vi "AOVoltageDAQmxGenWaveformBufferGeneration.vi"(0 "task/channels in":refnum<k21>, 1 "Samples per Buffer":dbl=1000.0, 3 "Amplitude":dbl=2.0 format="%0.2p", 5 "Desired Frequency":dbl=1000.0 format="%.2f", 7 "Waveform Type":T1(ring), 11 "error in (no error)":errorcluster, 12 "Cycles per Buffer":dbl=1.0 format="%.2f", 13 "Offset":dbl format="%0.2p") -> (4 "task out":refnum<k21>, 6 "Waveform":waveform(dbl), 10 "Resulting Frequency":dbl format="%.2f", 14 "Resulting Sample Clock Rate":dbl format="%.2f", 15 "error out":errorcluster)   [LabVIEW 2012]
doc: "This subVI is used to create a Sine, Square, Triangle or Sawtooth Waveform. The inputs to this VI are the Waveform Type, which determines if the output waveform is a Sine, Square, Triangle, or Sawtooth Waveform, the amplitude, Desired Frequency, Samples per Buffer, and Cycles per Buffer. \n\nThe Desired Frequency, Samples per Buffer, and Cycles per Buffer are used to calculate the sample clock rate. The DAQmx Timing property node sets the sample clock rate for the device specified in the task/channels in control. \n\nThe actual, coerced, sample clock rate is returned and used as an input to the Basic Function Generator.vi. The Basic Function Generator returns a waveform of data with timing information.\n\nThe formula below was used to determine the sample clock rate:\n\nDesired Frequency=[(Cycles/Buffer)X(Sample Clock Rate)]/Samples per Buffer\n\nNote: The Block Diagram rearranges the variables to solve for Sample Clock Rate"
uses:
  <vilib>/measure/NI_MABase.lvlib
  <resource>/objmgr/daqmx.rc
panel:
  out "Samples/cycle":dbl format="%0.2f"
  out "Desired Sample Clock Rate":dbl format="%.2f"
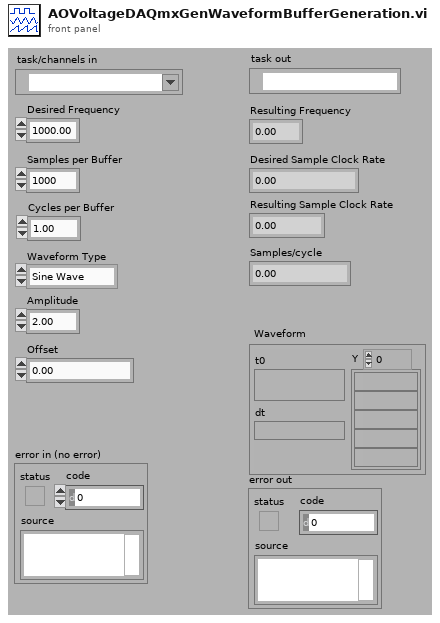
[diagram p1: front panel]
types:
  T1 = enum16{"Sine Wave", "Triangle Wave", "Square Wave", "Sawtooth Wave"}
  T2 = cluster{"SampClk.Rate":dbl, "Samples per Buffer":dbl}
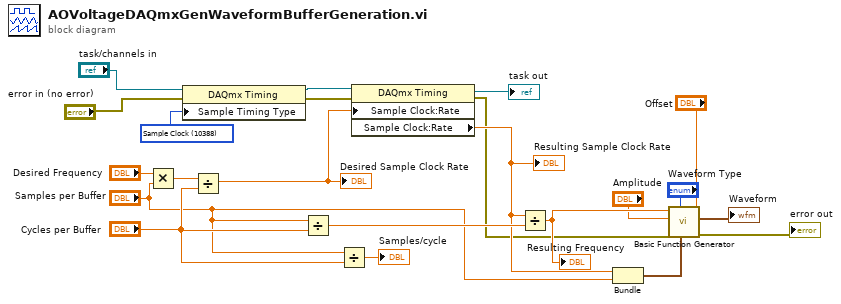
[diagram p0: block diagram]
diagram:
  w4 = 10388 items=["Sample Clock"=10388, "Handshake"=10389, "Implicit"=10451, "On Demand"=10390, "Change Detection"=12504] ("SampTimingType")
  n1 = Multiply(x="Desired Frequency", y="Samples per Buffer") -> (x*y=w18:dbl)
  n2 = property class="DAQmx Timing"(reference="task/channels in", error in="error in (no error)", "Sample Timing Type"=w4) -> (reference out=w6:refnum<k21>, error out=w5:errorcluster)
  n3 = Divide(x=w18, y="Cycles per Buffer") -> (x/y=w14:dbl)
  "Desired Sample Clock Rate" <- w14
  n4 = Divide(x="Samples per Buffer", y="Cycles per Buffer") -> (x/y=w15:dbl)
  n5 = Divide(x="Samples per Buffer", y="Cycles per Buffer") -> (x/y=→"Samples/cycle":dbl)
  n6 = property class="DAQmx Timing"(reference=w6, error in=w5, "Sample Clock:Rate"=w14) -> (reference out=→"task out":refnum<k21>, error out=w8:errorcluster, "Sample Clock:Rate"=w9:dbl)
  "Resulting Sample Clock Rate" <- w9
  n7 = Divide(x=w9, y=w15) -> (x/y=w22:dbl)
  "Resulting Frequency" <- w22
  n8 = Bundle("SampClk.Rate"=w9, "Samples per Buffer"="Samples per Buffer") -> (w20:T2)  [unwired: 1 in]
  n9 = call <vilib>:"Basic Function Generator.vi"("offset"="Offset", "sampling info"=w20, "signal type"="Waveform Type", "error in (no error)"=w8, "amplitude"="Amplitude", "frequency"=w22) -> ("error out"=→"error out":errorcluster, "signal out"=→"Waveform":waveform(dbl))  [unwired: 3 in, 1 out]
